vi "fg_temp_dir_config.vi"(8 "error in (no error)":errorcluster) -> (0 "error out":errorcluster, 3 "temp_dir_config out":T1)   [LabVIEW 2015, in "lv-bin-7zip.lvlib"]
uses:
  lv-bin-7zip.lvlib
  <userlib>/antonio-alexander/lv-bin/lv-bin/public/api/v1/_controls/temp_dir_config.ctl
  <vilib>/Utility/sysdir.llb/System Directory Type.ctl
  <userlib>/antonio-alexander/lv-bin/lv-bin/public/api/v1/v1.lvlib
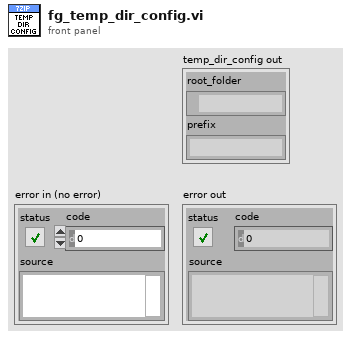
[diagram p1: front panel]
types:
  T1 = typedef "lv-bin.lvlib/v1.lvlib/temp_dir_config.ctl" = cluster{"root_folder":path, "prefix":string}
  T2 = typedef "System Directory Type.ctl" = i32
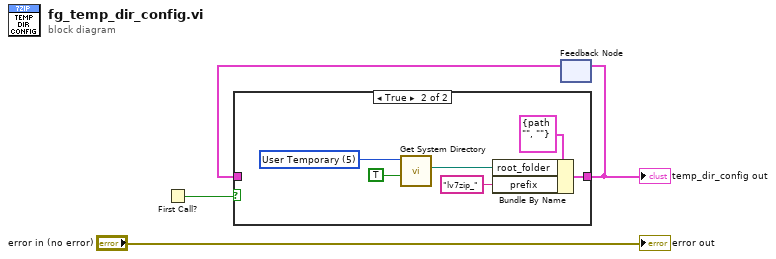
[diagram p0: block diagram]
diagram:
  n1 = First Call?() -> (First Call?: T/F=w3:bool)
  n2 = feedback #1() -> (w1:T1)  [unwired: 1 in]
  n3 = case shown="True" w3 {
    tunnel: [w5 w10] -> w2
    tunnel: w1 -> [w5 _]
    frame False {
    }
    frame True {
      w9 = T2 5 items=["User Home"=0, "User Desktop"=1, "User Documents"=2, "User Application Data"=3, "User Preferences"=4, "User Temporary"=5, "Public Documents"=6, "Public Application Data"=7, "Public Preferences"=8, "Public Cache"=13, "System Core Libraries"=9, "System Installed Libraries"=10, "Application Files"=11, "Boot Volume Root"=12] ("system directory type")
      n4 = call <vilib>:"Get System Directory.vi"("create directory if not found? (F)"=TRUE, "system directory type"=w9) -> ("system directory"=w7:path)  [unwired: 9 in]
      n5 = Bundle By Name(cluster=T1 {"root_folder"=path "", "prefix"=""} ("temp_dir_config out"), "root_folder"=w7, "prefix"="lv7zip_") -> (w10:T1)
    }
  }
  "temp_dir_config out" <- w2
  n6 = feedback-in #1(w2) -> ()
  "error out" <- "error in (no error)"
